vi "FTW-Connector-SpawnNewActor.vi"(0 "FTW Actor Connector Type":refnum<class "FTW-ActorConnector.lvclass">, 5 "Instance Configuration":string="{\n  \"Identity\": \"ActorName\",\n  \"InboxAddress\": \"tcp://127.0.0.1:*\",\n  \"PublisherAddress\": \"tcp://127.0.0.1:*\",\n  \"DebugEnableInboxLogging\": false,\n  \"DebugEnableJobLogging\": false,\n  \"DebugShowPanel\": false\n}", 7 "Timeout":i32=1000 format="%dmsec", 11 "error in":errorcluster) -> (4 "FTW Actor Connector":refnum<class "FTW-ActorConnector.lvclass">, 6 "Initialized Response":string, 8 "Instance Inbox Address":string, 10 "Instance Publisher Address":string, 15 "error out":errorcluster)   [LabVIEW 2012, in "FTW-Actor.lvlib" / "FTW-ActorConnector.lvclass"]
uses:
  FTW-ActorConnector.lvclass
  Endpoint/FTW-Endpoint-Type.ctl
  Endpoint/FTW-Endpoint.lvclass
panel:
  # "Inputs"
  # "Outputs"
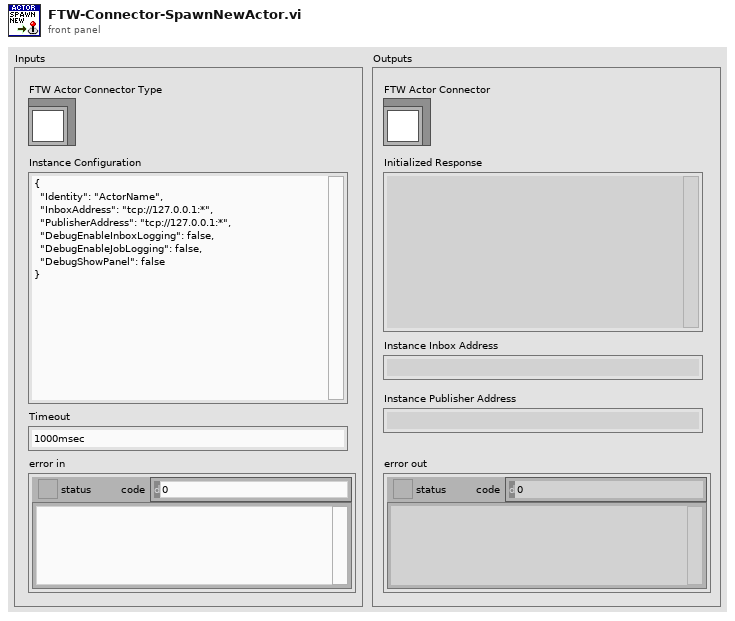
[diagram p1: front panel]
types:
  T1 = typedef "FTW-Actor.lvlib/FTW-Endpoint.lvclass/FTW-Endpoint-Type.ctl" = enum32{"Server", "Client", "Publisher", "Subscriber", "Pipeline Producer", "Pipeline Consumer", "Surveyor", "Respondent", "Exclusive Pair", "Bus"}
  T2 = cluster{"InboxAddress":string, "PublisherAddress":string}
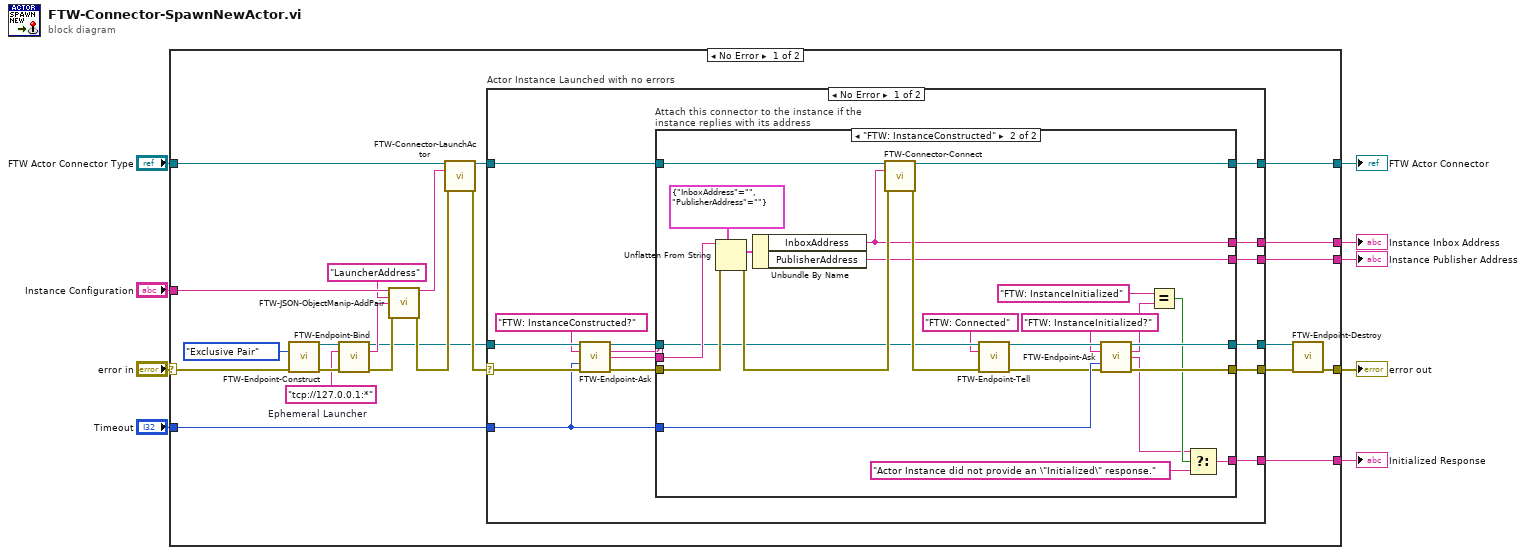
[diagram p0: block diagram]
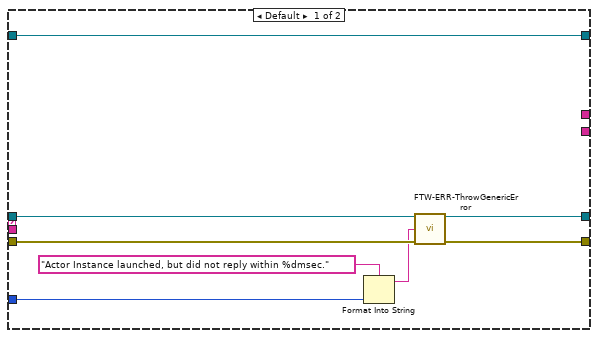
[diagram p2: hidden frame]
diagram:
  n1 = case shown="No Error" "error in" {
    selector: "error in" -> [w14 w83]
    tunnel: [w26 w83] -> w4
    tunnel: [w32 w82] -> w5
    tunnel: "FTW Actor Connector Type" -> [w25 w82]
    tunnel: "Instance Configuration" -> [w31 _]
    tunnel: "Timeout" -> [w29 _]
    tunnel: [w21 _] -> w3
    tunnel: [w20 _] -> w2
    tunnel: [w19 _] -> w1
    frame No Error {
      w16 = "tcp://127.0.0.1:*"  # Ephemeral Launcher
      n2 = call "FTW-Endpoint-Construct.vi"("Socket Type"=FTW-Endpoint-Type."Exclusive Pair", "error in"=w14) -> ("FTW Socket"=w18:refnum<class "FTW-Endpoint.lvclass">, "error out"=w17:errorcluster)  [unwired: 12 in]
      n3 = call-dynamic "FTW-Endpoint-Bind.vi"("FTW Socket"=w18, "Endpoint Address"=w16, "error in"=w17) -> ("FTW Socket out"=w11:refnum<class "FTW-Endpoint.lvclass">, "Actual Endpoint Address"=w13:string, "error out"=w12:errorcluster)  [unwired: 9 in, 1 out]
      n4 = call "FTW-JSON-ObjectManip-AddPair.vi"("Input JSON Object"=w31, "Key"="LauncherAddress", "Value"=w13, "error in"=w12) -> ("Output JSON Object"=w10:string, "error out"=w23:errorcluster)  [unwired: 10 in]
      n5 = call-dynamic "FTW-Connector-LaunchActor.vi"("FTW Actor Connector"=w25, "Actor Instance Configuration"=w10, "error in"=w23) -> ("FTW Actor Connector out"=w24:refnum<class "FTW-ActorConnector.lvclass">, "error out"=w22:errorcluster)  [unwired: 11 in]
      n6 = case "Actor Instance Launched with no errors" shown="No Error" w22 {
        selector: w22 -> [w42 w80]
        tunnel: [w47 w80] -> w27
        tunnel: w24 -> [w46 w81]
        tunnel: [w45 w81] -> w32
        tunnel: w11 -> [w43 w79]
        tunnel: w29 -> [w41 _]
        tunnel: [w44 w79] -> w28
        tunnel: [w38 _] -> w21
        tunnel: [w37 _] -> w20
        tunnel: [w36 _] -> w19
        frame No Error {
          n7 = call-dynamic "FTW-Endpoint-Ask.vi"("FTW Socket"=w43, "Request Header"="FTW: InstanceConstructed?", "Timeout"=w41, "error in"=w42) -> ("FTW Socket out"=w39:refnum<class "FTW-Endpoint.lvclass">, "Response Header"=w34:string, "Response Body"=w33:string, "error out"=w40:errorcluster)  [unwired: 7 in, 1 out]
          n8 = case "Attach this connector to the instance if the instance replies with its address" shown="\"FTW: InstanceConstructed\"" w34 {
            tunnel: [w52 w74] -> w47
            tunnel: w46 -> [w54 w77]
            tunnel: [w54 w76] -> w45
            tunnel: w39 -> [w51 w56]
            tunnel: w40 -> [w53 w62]
            tunnel: [w51 w75] -> w44
            tunnel: w41 -> [w49 w67]
            tunnel: [_ w68] -> w38
            tunnel: [_ w58] -> w37
            tunnel: [_ w59] -> w36
            tunnel: w33 -> [_ w63]
            frame Default {
              n9 = Format Into String(format string="Actor Instance launched, but did not reply within %dmsec." ("Error Message"), w49) -> (resulting string=w48:string)  [unwired: 2 in, 1 out]
              n10 = call "FTW-ERR-ThrowGenericError.vi"("Error Message"=w48, "error in"=w53) -> ("error out"=w52:errorcluster)  [unwired: 13 in]
            }
            frame "FTW: InstanceConstructed" {
              n11 = Unflatten From String(type=T2 {"InboxAddress"="", "PublisherAddress"=""}, binary string=w63, error in (no error)=w62) -> (value=w60:T2, error out=w61:errorcluster)  [unwired: 2 in, 1 out]
              n12 = Unbundle By Name(w60) -> ("InboxAddress"=w59:string, "PublisherAddress"=w58:string)
              n13 = call-dynamic "FTW-Connector-Connect.vi"("FTW Actor Connector Type"=w77, "Instance Inbox Address"=w59, "error in"=w61) -> ("FTW Actor Connector"=w76:refnum<class "FTW-ActorConnector.lvclass">, "error out"=w78:errorcluster)  [unwired: 11 in]
              n14 = call-dynamic "FTW-Endpoint-Tell.vi"("FTW Socket"=w56, "Message Header"="FTW: Connected", "error in"=w78) -> ("FTW Socket out"=w66:refnum<class "FTW-Endpoint.lvclass">, "error out"=w65:errorcluster)  [unwired: 10 in, 1 out]
              n15 = call-dynamic "FTW-Endpoint-Ask.vi"("FTW Socket"=w66, "Request Header"="FTW: InstanceInitialized?", "Timeout"=w67, "error in"=w65) -> ("FTW Socket out"=w75:refnum<class "FTW-Endpoint.lvclass">, "Response Header"=w72:string, "Response Body"=w70:string, "error out"=w74:errorcluster)  [unwired: 7 in, 1 out]
              n16 = Equal?(x="FTW: InstanceInitialized", y=w72) -> (x = y?=w71:bool)
              n17 = Select(t=w70, s=w71, f="Actor Instance did not provide an \"Initialized\" response.") -> (s? t:f=w68:string)
            }
          }
        }
        frame Error {
        }
      }
      n18 = call-dynamic "FTW-Endpoint-Destroy.vi"("FTW Socket"=w28, "error in"=w27) -> ("error out"=w26:errorcluster)  [unwired: 13 in]
    }
    frame Error {
    }
  }
  "error out" <- w4
  "FTW Actor Connector" <- w5
  "Initialized Response" <- w3
  "Instance Inbox Address" <- w1
  "Instance Publisher Address" <- w2
